vi "Straight Movement.vi"(9 "EncoderDevRef":T11={"DevStatus"={"status"=FALSE, "code"=0, "source"=""}, "EncoderIndex"=enum."Invalid", "CounterIndex"=enum."Ctr 1", "DistancePerCount"=2.0, "Decoding Type"=enum."4x"}, 10 "EncoderDevRef 2":T11={"DevStatus"={"status"=FALSE, "code"=0, "source"=""}, "EncoderIndex"=enum."Invalid", "CounterIndex"=enum."Ctr 1", "DistancePerCount"=2.0, "Decoding Type"=enum."4x"}, 11 "RobotDriveDevRef":T3={"DevStatus"={"status"=FALSE, "code"=0, "source"=""}, "Motors[]"=[], "Square Inputs"=FALSE, "Max Output"=1.0, "Isochronous"=FALSE}) -> (3 "Finished?":bool)   [LabVIEW 2012]
uses:
  <vilib>/addons/control/pid/NI_PID_pid.lvlib
  <vilib>/addons/control/pid/pid.llb/PID (DBL).vi
  <vilib>/Rock Robotics/SystemInterfaces/Encoder/FPGA_EncoderIdx.ctl
  <vilib>/Rock Robotics/WPI/Encoder/WPI_EncoderType.ctl
  <vilib>/Rock Robotics/SystemInterfaces/Counter/FPGA_CounterCtrSystemIndex.ctl
  <vilib>/Rock Robotics/WPI/Encoder/WPI_EncoderDevRef.ctl
  <vilib>/Rock Robotics/WPI/PWM/WPI_PWMTransform_ConPane.ctl
  <vilib>/Rock Robotics/SystemInterfaces/Typedef/FPGA_TypedefDigitalModule.ctl
  <vilib>/Rock Robotics/SystemInterfaces/DIO/FPGA_DIOPWMChannel.ctl
  <vilib>/Rock Robotics/WPI/PWM/WPI_PWMDeadband.ctl
  <vilib>/Rock Robotics/WPI/CAN/Jaguar/SubVIs/WPI_CANJaguar_ControlMode.ctl
  <vilib>/Rock Robotics/WPI/MotorControl/WPI_MotorControlDeviceRef.ctl
  <vilib>/Rock Robotics/WPI/RobotDrive/WPI_RobotDriveDevRef.ctl
panel:
  in  "Spare Correction Time":dbl
  in  "Times":T1
  in  "Tolerance":dbl
  in  "PID gains":T2={"proportional gain (Kc)"=1.0, "integral time (Ti, min)"=0.01, "derivative time (Td, min)"=0.0} {"derivative time (Td, min)" format="%.3f"; "integral time (Ti, min)" format="%.3f"; "proportional gain (Kc)" format="%.3f"}
  in  "Correction PID gains":T2={"proportional gain (Kc)"=1.0, "integral time (Ti, min)"=0.01, "derivative time (Td, min)"=0.0} {"derivative time (Td, min)" format="%.3f"; "integral time (Ti, min)" format="%.3f"; "proportional gain (Kc)" format="%.3f"}
  in  "Distance to Move":dbl
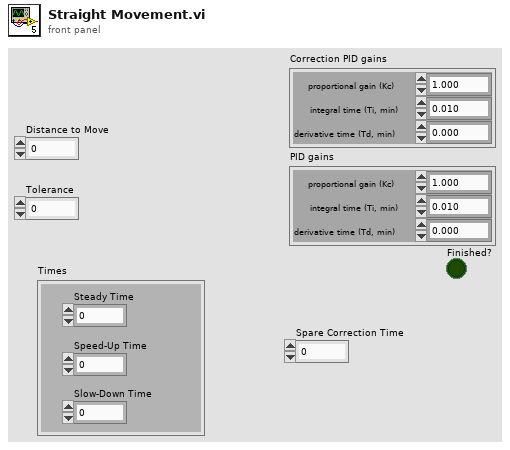
[diagram p1: front panel]
types:
  T1 = cluster{"Steady Time":dbl, "Speed-Up Time":dbl, "Slow-Down Time":dbl}
  T2 = cluster{"proportional gain (Kc)":dbl, "integral time (Ti, min)":dbl, "derivative time (Td, min)":dbl}
  T3 = typedef "WPI_RobotDriveDevRef.ctl" = cluster{"DevStatus":errorcluster, "Motors[]":T4[], "Square Inputs":bool, "Max Output":dbl, "Isochronous":bool}
  T4 = typedef "WPI_MotorControlDeviceRef.ctl" = cluster{"DeviceStatus":errorcluster, "Type":enum16{"PWM", "CAN"}, "PWM":cluster{"Digital Module":T5, "PWM Channel":T6, "DeadBand":T7}, "CAN":cluster{"Device Number":u8, "Control Mode":T8, "Semaphore":T9, "Max Vout":dbl}, "Invert":bool, "TransformRef":T10, "InvTransformRef":T10}
  T5 = typedef "FPGA_TypedefDigitalModule.ctl" = enum16{"Digital Module 1", "Digital Module 2"}
  T6 = typedef "FPGA_DIOPWMChannel.ctl" = enum8{"PWM 1", "PWM 2", "PWM 3", "PWM 4", "PWM 5", "PWM 6", "PWM 7", "PWM 8", "PWM 9", "PWM 10", "Invalid"}
  T7 = typedef "WPI_PWMDeadband.ctl" = cluster{"Name":string, "maxPositivePwm":i32, "minPositivePwm":i32, "centerPwm":i32, "maxNegativePwm":i32, "minNegativePwm":i32, "angularRange":u16}
  T8 = typedef "WPI_CANJaguar_ControlMode.ctl" = enum8{"Percent VBus", "Current", "Speed", "Position", "Voltage"}
  T9 = typedef "Semaphore RefNum" = refnum<k1>
  T10 = typedef "WPI_PWMTransform_ConPane.ctl" = refnum<vi>
  T11 = typedef "WPI_EncoderDevRef.ctl" = cluster{"DevStatus":errorcluster, "EncoderIndex":T12, "CounterIndex":T13, "DistancePerCount":dbl, "Decoding Type":T14}
  T12 = typedef "FPGA_EncoderIdx.ctl" = enum8{"Enc 0", "Enc 1", "Enc 2", "Enc 3", "Invalid"}
  T13 = typedef "FPGA_CounterCtrSystemIndex.ctl" = enum8{"Ctr 0", "Ctr 1", "Ctr 2", "Ctr 3", "Ctr 4", "Ctr 5", "Ctr 6", "Ctr 7", "Invalid"}
  T14 = typedef "WPI_EncoderType.ctl" = enum16{"1x", "2x", "4x"}
  T15 = cluster{"Speed-Up Time":dbl, dbl, "Slow-Down Time":dbl}
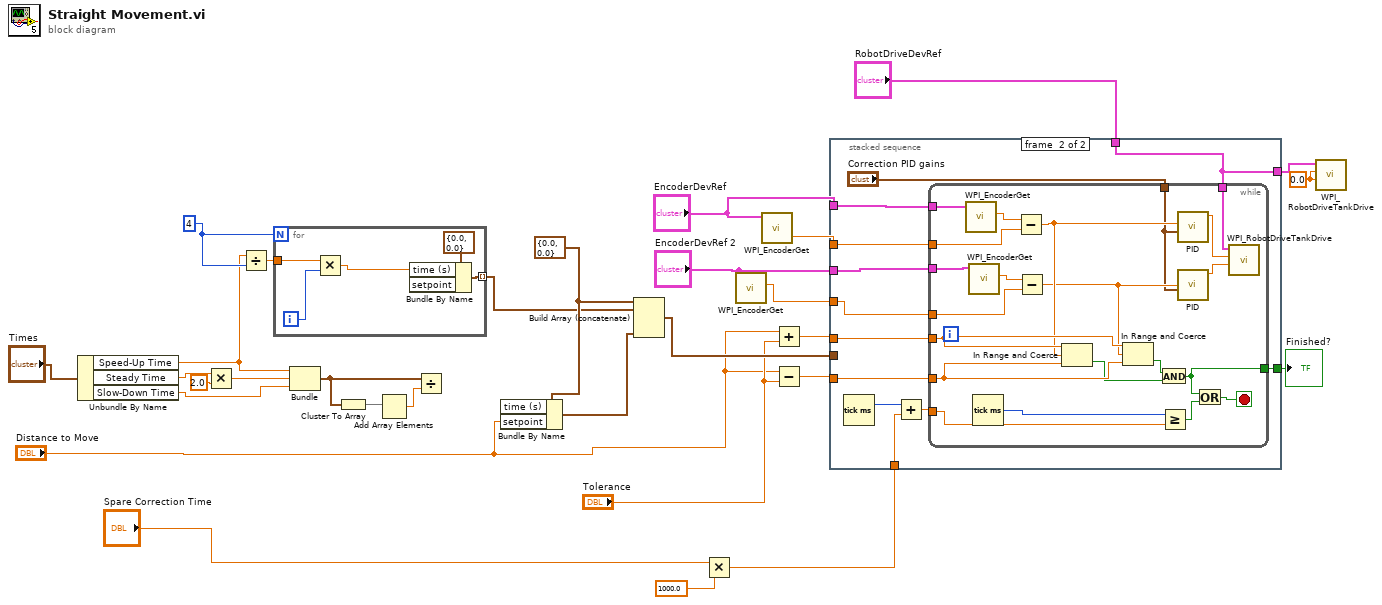
[diagram p0: block diagram]
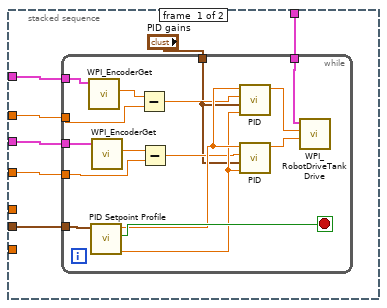
[diagram p2: hidden frame]
diagram:
  w11 = 4
  w16 = 0.0 ("Left axis value")
  w30 = cluster{"time (s)":dbl, "setpoint":dbl} {"time (s)"=0.0, "setpoint"=0.0}
  n1 = Unbundle By Name("Times") -> ("Speed-Up Time"=w6:dbl, "Steady Time"=w8:dbl, "Slow-Down Time"=w4:dbl)
  n2 = Multiply(x=w8, y=2.0) -> (x*y=w5:dbl)
  n3 = Divide(x=w6, y=w11) -> (x/y=w10:dbl)
  n4 = for {
    N: w11 -> [_]
    tunnel: [w34] -> w12 mode=indexing
    tunnel: w10 -> [w32]
    i -> [w33]
    n5 = Multiply(x=w32, y=w33) -> (x*y=w31:dbl)
    n6 = Bundle By Name(cluster=cluster{"time (s)":dbl, "setpoint":dbl} {"time (s)"=0.0, "setpoint"=0.0}, "time (s)"=w31) -> (w34:cluster{"time (s)":dbl, "setpoint":dbl})  [unwired: 1 in]
  }
  n7 = Bundle("Speed-Up Time"=w6, w5, "Slow-Down Time"=w4) -> (w1:T15)  [unwired: 1 in]
  n8 = Cluster To Array(cluster=w1) -> (array=w3:dbl[])
  n9 = Add Array Elements(numeric array=w3) -> (sum=w2:dbl)
  n10 = Divide(x=w1, y=w2) -> ()  [unwired: 1 out]
  n11 = Bundle By Name(cluster=w30, "setpoint"="Distance to Move") -> (w13:cluster{"time (s)":dbl, "setpoint":dbl})  [unwired: 1 in]
  n12 = Build Array (concatenate)(w30, w12, w13) -> (w29:cluster{"time (s)":dbl, "setpoint":dbl}[])  [unwired: 2 in]
  n13 = Multiply(x="Spare Correction Time", y=1000.0) -> (x*y=w21:dbl)
  n14 = call <vilib>:"WPI_EncoderGet.vi"("EncoderDevRef"="EncoderDevRef 2") -> ("Distance"=w27:dbl)  [unwired: 5 in, 5 out]
  n15 = call <vilib>:"WPI_EncoderGet.vi"("EncoderDevRef"="EncoderDevRef") -> ("Distance"=w28:dbl)  [unwired: 5 in, 5 out]
  n16 = Add(x="Distance to Move", y="Tolerance") -> (x+y=w20:dbl)
  n17 = Subtract(x="Distance to Move", y="Tolerance") -> (x-y=w19:dbl)
  n18 = stacked-sequence {
    tunnel: w29 -> [w42 _]
    tunnel: "EncoderDevRef 2" -> [w41 w66]
    tunnel: "EncoderDevRef" -> [w40 w67]
    tunnel: w28 -> [w39 w65]
    tunnel: w27 -> [w38 w64]
    tunnel: "RobotDriveDevRef" -> [w36 w59]
    tunnel: w21 -> [_ w69]
    tunnel: w20 -> [_ w63]
    tunnel: w19 -> [_ w62]
    tunnel: [_ w60] -> w17
    tunnel: [_ w59] -> w15
    frame #0 {
      n19 = while {
        tunnel: w42 -> [w55]
        tunnel: w41 -> [w50]
        tunnel: w40 -> [w54]
        tunnel: w39 -> [w52]
        tunnel: w38 -> [w49]
        tunnel: w36 -> [w44]
        tunnel: "PID gains" -> [w43]
        stop <- w58 stop-if-true
        n20 = call <vilib>:"WPI_EncoderGet.vi"("EncoderDevRef"=w54) -> ("Distance"=w53:dbl)  [unwired: 5 in, 5 out]
        n21 = call <vilib>:"PID Setpoint Profile.vi"("setpoint profile"=w55) -> ("dt out (s)"=w56:dbl, "profile complete?"=w58:bool, "setpoint"=w57:dbl)  [unwired: 5 in, 1 out]
        n22 = call <vilib>:"WPI_EncoderGet.vi"("EncoderDevRef"=w50) -> ("Distance"=w48:dbl)  [unwired: 5 in, 5 out]
        n23 = Subtract(x=w53, y=w52) -> (x-y=w51:dbl)
        n24 = Subtract(x=w48, y=w49) -> (x-y=w47:dbl)
        n25 = call-poly <vilib>:"PID.vi"("dt (s)"=w56, "PID gains"=w43, "process variable"=w51, "setpoint"=w57) -> ("output"=w46:dbl)  [unwired: 6 in, 1 out]
        n26 = call-poly <vilib>:"PID.vi"("dt (s)"=w56, "PID gains"=w43, "process variable"=w47, "setpoint"=w57) -> ("output"=w45:dbl)  [unwired: 6 in, 1 out]
        n27 = call <vilib>:"WPI_RobotDriveTankDrive.vi"("Right axis value"=w45, "Left axis value"=w46, "RobotDriveDevRef"=w44) -> ()  [unwired: 6 in, 3 out]
      }
    }
    frame #1 {
      n28 = Tick Count (ms)() -> (millisecond timer value=w70:u32)
      n29 = Add(x=w70, y=w69) -> (x+y=w68:dbl)
      n30 = while {
        tunnel: w68 -> [w84]
        tunnel: w67 -> [w83]
        tunnel: w66 -> [w82]
        tunnel: w65 -> [w81]
        tunnel: w64 -> [w80]
        tunnel: w63 -> [w78]
        tunnel: w62 -> [w79]
        tunnel: "Correction PID gains" -> [w73]
        tunnel: w59 -> [w72]
        tunnel: [w71] -> w60
        stop <- w87 stop-if-true
        n31 = call <vilib>:"WPI_EncoderGet.vi"("EncoderDevRef"=w83) -> ("Distance"=w91:dbl)  [unwired: 5 in, 5 out]
        n32 = call <vilib>:"WPI_EncoderGet.vi"("EncoderDevRef"=w82) -> ("Distance"=w90:dbl)  [unwired: 5 in, 5 out]
        n33 = Tick Count (ms)() -> (millisecond timer value=w85:u32)
        n34 = Subtract(x=w91, y=w81) -> (x-y=w77:dbl)
        n35 = Subtract(x=w90, y=w80) -> (x-y=w76:dbl)
        n36 = In Range and Coerce(upper limit=w78, x=w77, lower limit=w79) -> (In Range?=w75:bool)  [unwired: 1 out]
        n37 = In Range and Coerce(upper limit=w78, x=w76, lower limit=w79) -> (In Range?=w74:bool)  [unwired: 1 out]
        n38 = And(x=w74, y=w75) -> (x .and. y?=w71:bool)
        n39 = Greater Or Equal?(x=w85, y=w84) -> (x >= y?=w86:bool)
        n40 = call-poly <vilib>:"PID.vi"("PID gains"=w73, "process variable"=w77) -> ("output"=w89:dbl)  [unwired: 8 in, 1 out]
        n41 = call-poly <vilib>:"PID.vi"("PID gains"=w73, "process variable"=w76) -> ("output"=w88:dbl)  [unwired: 8 in, 1 out]
        n42 = Or(x=w71, y=w86) -> (x .or. y?=w87:bool)
        n43 = call <vilib>:"WPI_RobotDriveTankDrive.vi"("Right axis value"=w88, "Left axis value"=w89, "RobotDriveDevRef"=w72) -> ()  [unwired: 6 in, 3 out]
      }
    }
  }
  "Finished?" <- w17
  n44 = call <vilib>:"WPI_RobotDriveTankDrive.vi"("Right axis value"=w16, "Left axis value"=w16, "RobotDriveDevRef"=w15) -> ()  [unwired: 6 in, 3 out]
